vi "DISP_FSIG.vi"(0 "VISA IN":refnum<visa-resource-name>, 5 "error in":errorcluster, 7 "ON | OFF":bool) -> (14 "VISA Out":refnum<visa-resource-name>, 19 "error out":errorcluster)   [LabVIEW 2018, in "PNA-X.lvlib"]
doc: "DISPlay:FSIGn <ON | OFF> \n(Read-Write) Shows or hides the window which displays global pass/fail results. \nParameters \n<ON | OFF> ON (or 1) - displays the pass/fail dialog \nOFF (or 0) - hides the pass/fail dialog \nExamples DISP:FSIG ON \ndisplay:fsign off \nQuery Syntax DISPlay:FSIGn? \nReturn Type Boolean (1 = ON, 0 = OFF) \nDefault OFF \nDISPlay[:TILE] - Superseded \n1589\n\nThis command is replaced by DISP:ARRange \n(Write-only) Tiles the windows on the screen. \nExamples DISP \ndisplay:tile \nDefault Not Applicable"
uses:
  PNA-X.lvlib
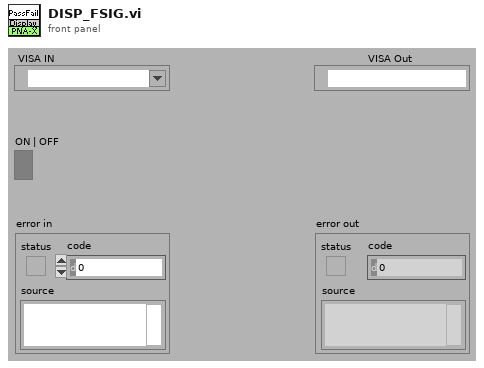
[diagram p1: front panel]
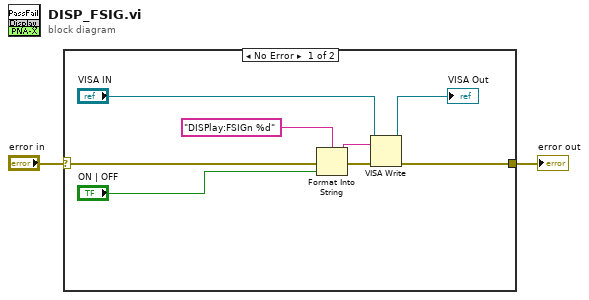
[diagram p0: block diagram]
diagram:
  n1 = case shown="No Error" "error in" {
    selector: "error in" -> [w10 w11]
    tunnel: [w5 w11] -> w1
    frame No Error {
      n2 = Format Into String(format string="DISPlay:FSIGn %d" ("Cmdline"), error in=w10, "ON | OFF") -> (resulting string=w8:string, error out=w9:errorcluster)  [unwired: 1 in]
      n3 = VISA Write(VISA resource name="VISA IN", write buffer=w8, error in (no error)=w9) -> (VISA resource name out=→"VISA Out":refnum<visa-resource-name>, error out=w5:errorcluster)  [unwired: 1 out]
    }
    frame Error {
    }
  }
  "error out" <- w1
